vi "serverLoop.vi"(8 "error in (no error)":errorcluster, 11 "tcpServer in":refnum<class "TcpServer.lvclass">) -> (0 "error out":errorcluster, 3 "tcpServer out":refnum<class "TcpServer.lvclass">)   [LabVIEW 2018, in "TcpServer.lvclass"]
doc: "Create TCP Listener and wait untill TcpClient starts. Then, authenticate the TcpClient and then start the readWritePacket.vi. When readWritePacket.vi ends, the TCP Listener connection ends too."
uses:
  TcpServer.lvclass
  TcpServer.lvclass/TcpServer.ctl
panel:
  out "Client IP":string
  out "loop":i32
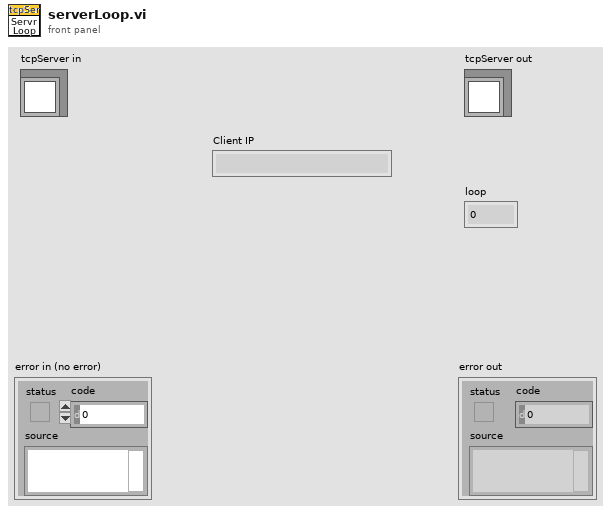
[diagram p1: front panel]
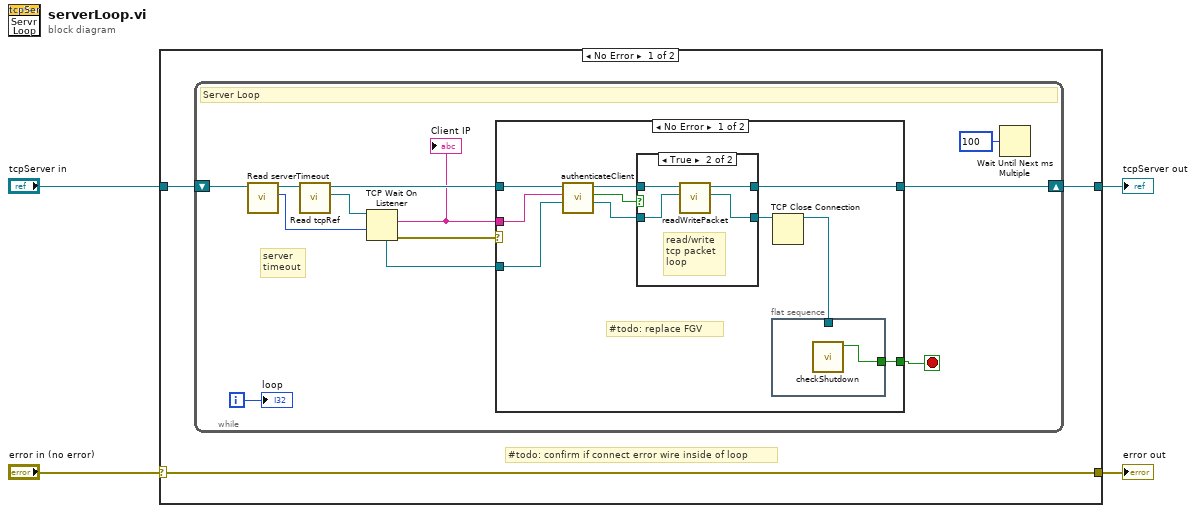
[diagram p0: block diagram]
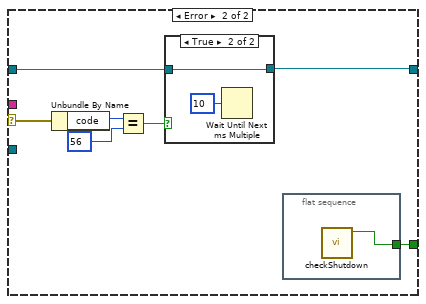
[diagram p3: hidden frame]
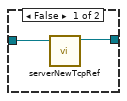
[diagram p4: hidden frame]
diagram:
  n1 = case shown="No Error" "error in (no error)" {
    selector: "error in (no error)" -> [w5 w50]
    tunnel: [w5 w50] -> w3
    tunnel: [w6 w49] -> w1
    tunnel: "tcpServer in" -> [w7 w49]
    frame No Error {
      # "#todo: confirm if connect error wire inside of loop"
      n2 = while {
        shift-right: [w14] -> w6
        shift-left: w7 -> [w8]
        i -> [w13]
        stop <- w12 stop-if-true
        # "server\ntimeout"
        # "Server Loop"
        n3 = call "Read serverTimeout.vi"("tcpServer in"=w8) -> ("serverTimeout"=w9:i32, "tcpServer out"=w10:refnum<class "TcpServer.lvclass">)  [unwired: 8 in, 1 out]
        n4 = call "Read tcpRef.vi"("tcpServer in"=w10) -> ("tcpRef"=w19:refnum<k5>, "tcpServer out"=w18:refnum<class "TcpServer.lvclass">)  [unwired: 8 in, 1 out]
        n5 = TCP Wait On Listener(9:w9, 11:w19) -> (0:w17:errorcluster, 2:w11:string, 4:w16:refnum<k5>)  [unwired: 2 in, 2 out]
        "Client IP" <- w11
        n6 = case shown="No Error" w17 {
          selector: w17 -> [_ w41]
          tunnel: w18 -> [w29 w39]
          tunnel: w16 -> [w28 _]
          tunnel: [w23 w38] -> w14
          tunnel: [w22 w37] -> w12
          tunnel: w11 -> [w20 _]
          frame No Error {
            # "#todo: replace FGV"
            n7 = call "authenticateClient.vi"("connection ID"=w28, "Computer Name"=w20, "tcpServer in"=w29) -> ("connection ID"=w25:refnum<k5>, "authenticate"=w27:bool, "tcpServer out"=w26:refnum<class "TcpServer.lvclass">)  [unwired: 5 in, 1 out]
            n8 = case shown="True" w27 {
              tunnel: w26 -> [w31 w36]
              tunnel: w25 -> [w32 w35]
              tunnel: [w32 w34] -> w24
              tunnel: [w31 w33] -> w23
              frame False {
                # "close connection\nif  authenticattion\nfailed."
              }
              frame True {
                # "read/write\ntcp packet \nloop"
                n9 = call "readWritePacket.vi"("tcpRef"=w35, "tcpServer in"=w36) -> ("tcpRef"=w34:refnum<k5>, "tcpServer out"=w33:refnum<class "TcpServer.lvclass">)  [unwired: 7 in, 1 out]
              }
            }
            n10 = flat-sequence {
              tunnel: [w30] -> w22
              tunnel: w21 -> [_]
              frame #0 {
                n11 = call "checkShutdown.vi"() -> ("shutdown?"=w30:bool)  [unwired: 10 in, 1 out]
              }
            }
            n12 = TCP Close Connection(connection ID=w24) -> (connection ID out=w21:refnum<k5>)  [unwired: 2 in, 1 out]
          }
          frame Error {
            n13 = Unbundle By Name(w41) -> ("code"=w43:i32)
            n14 = Equal?(x=w43, y=56) -> (x = y?=w40:bool)
            n15 = case shown="True" w40 {
              tunnel: w39 -> [w46 w47]
              tunnel: [w45 w47] -> w38
              frame False {
                n16 = call "serverNewTcpRef.vi"("tcpServer in"=w46) -> ("tcpServer out"=w45:refnum<class "TcpServer.lvclass">)  [unwired: 9 in, 1 out]
              }
              frame True {
                n17 = Wait Until Next ms Multiple(millisecond multiple=u32 10) -> ()  [unwired: 1 out]
              }
            }
            n18 = flat-sequence {
              tunnel: [w44] -> w37
              frame #0 {
                n19 = call "checkShutdown.vi"() -> ("shutdown?"=w44:bool)  [unwired: 10 in, 1 out]
              }
            }
          }
        }
        n20 = Wait Until Next ms Multiple(millisecond multiple=u32 100) -> ()  [unwired: 1 out]
        "loop" <- w13
      }
    }
    frame Error {
    }
  }
  "error out" <- w3
  "tcpServer out" <- w1
